vi "Stop_Item.vi"(8 "error in (no error)":errorcluster, 10 "Index":i32, 11 "Item_Refnums_Array":T1[](array[typedef])) -> (0 "error out":errorcluster, 3 "Item_Refnums_Array Out":T1[](array[typedef]))   [LabVIEW 2011, in "Root_XControl.xctl"]
uses:
  Root_XControl.xctl
  Controls/References/Item_Refnums.ctl
  Controls/References/Item_Command_Refnum.ctl
  Controls/Item_Command_Enum.ctl
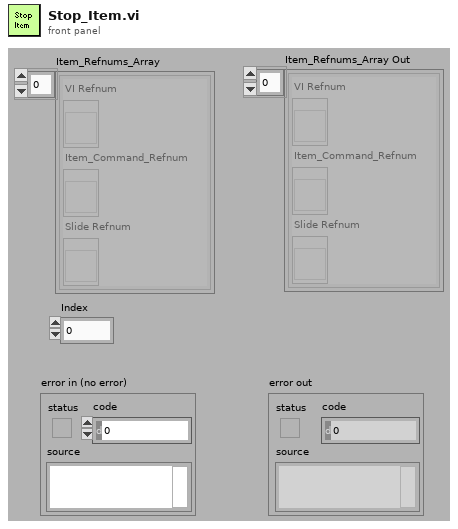
[diagram p1: front panel]
types:
  T1 = typedef "Item_Refnums.ctl" = cluster{"VI Refnum":refnum<vi>, "Item_Command_Refnum":T2, "Slide Refnum":refnum<vi>}
  T2 = typedef "Item_Command_Refnum.ctl" = refnum<vi>
  T3 = typedef "Item_Command_Enum.ctl" = enum16{"Stop", "Insert into Subpanel", "Update Value", "Remove from Subpanel"}
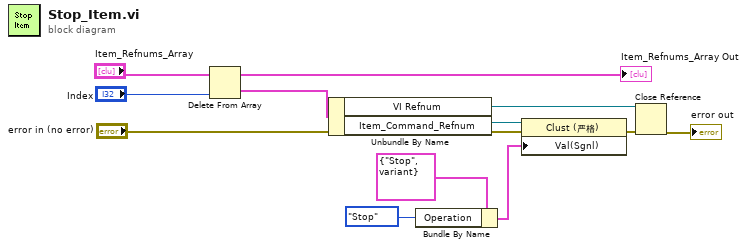
[diagram p0: block diagram]
diagram:
  n1 = Delete From Array "Delete From Array"(array="Item_Refnums_Array", index="Index") -> (deleted portion=w6:T1, array with subset deleted=→"Item_Refnums_Array Out":T1[])  [unwired: 1 in]
  n2 = Unbundle By Name(w6) -> ("VI Refnum"=w11:refnum<vi>, "Item_Command_Refnum"=w7:T2)
  n3 = Bundle By Name(cluster=cluster{"Operation":T3, "Data":variant} {"Operation"=enum."Stop", "Data"=variant} ("Item_Command"), "Operation"=Item_Command_Enum."Stop") -> (w10:cluster{"Operation":T3, "Data":variant})
  n4 = property class="Clust (严格)"(reference=w7, error in="error in (no error)", "Val(Sgnl)"=w10) -> (error out=w12:errorcluster)  [unwired: 1 out]
  n5 = Close Reference(reference=w11, error in (no error)=w12) -> (error out=→"error out":errorcluster)
